vi "GFITS_ImlistMngr.vi"(6 "max bytes size":i32=200000, 8 "log":bool, 9 "arguments":string, 10 "command":string, 11 "images_witten_path":path=path "/home/ArcVIEW/Modules/Database/private/vis/imlist.log") -> (0 "log out":bool, 2 "answer":string)   [LabVIEW 2016]
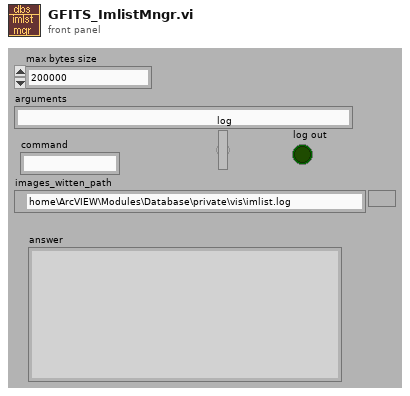
[diagram p1: front panel]
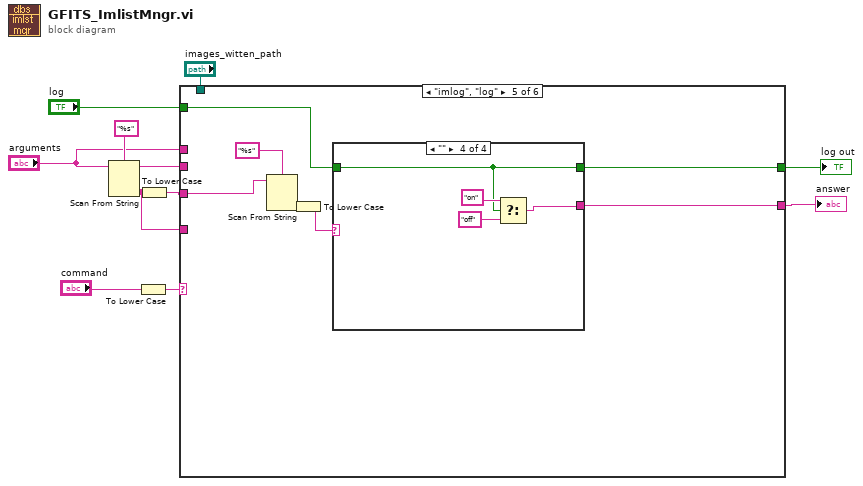
[diagram p0: block diagram]
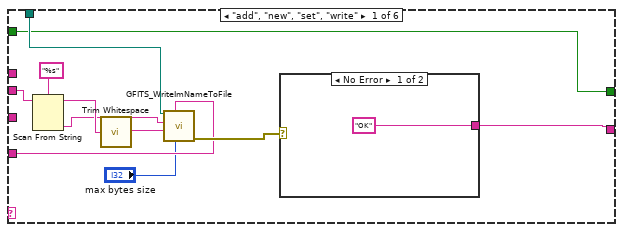
[diagram p2: hidden frame]
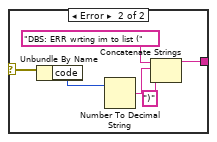
[diagram p3: hidden frame]
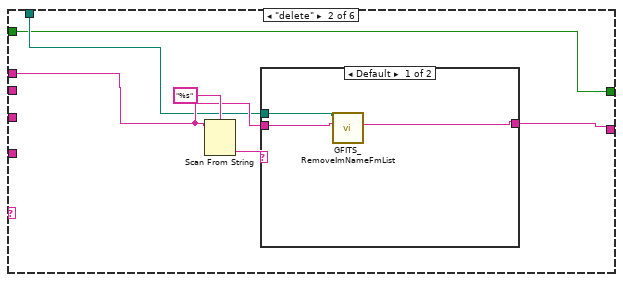
[diagram p4: hidden frame]
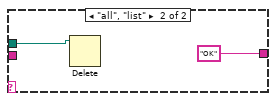
[diagram p5: hidden frame]
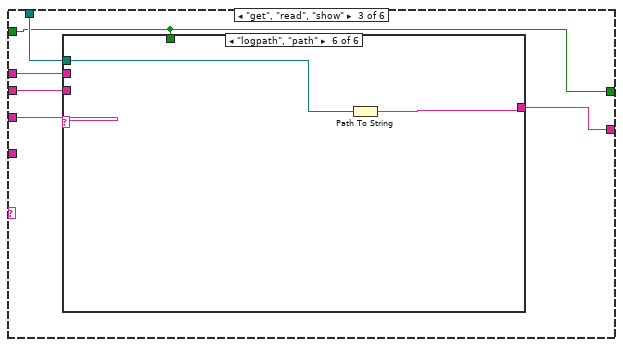
[diagram p6: hidden frame]
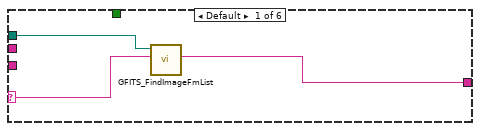
[diagram p7: hidden frame]
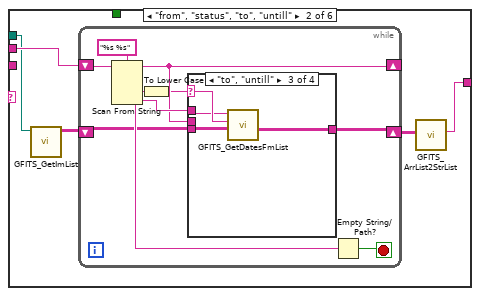
[diagram p8: hidden frame]
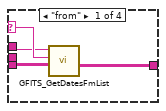
[diagram p9: hidden frame]
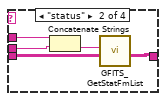
[diagram p10: hidden frame]
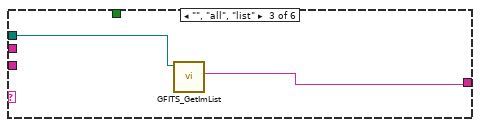
[diagram p12: hidden frame]
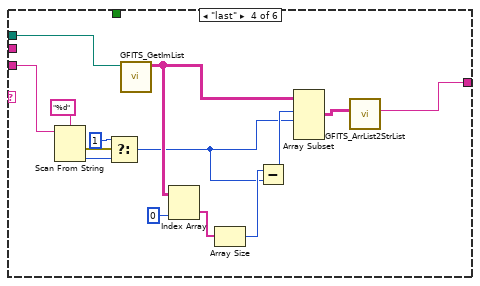
[diagram p13: hidden frame]
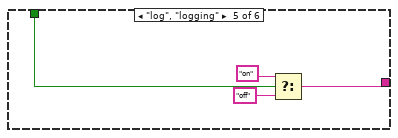
[diagram p14: hidden frame]
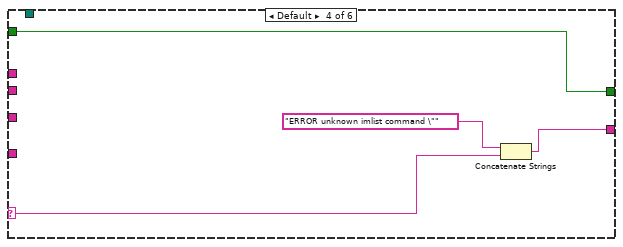
[diagram p15: hidden frame]
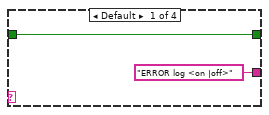
[diagram p16: hidden frame]
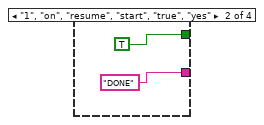
[diagram p17: hidden frame]
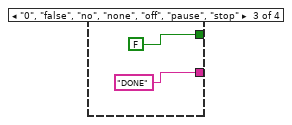
[diagram p18: hidden frame]
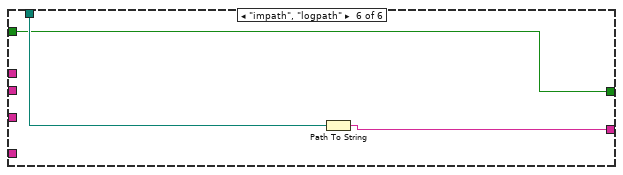
[diagram p19: hidden frame]
diagram:
  n1 = Scan From String(format string="%s", input string="arguments") -> (remaining string=w10:string, output 1=w3:string)  [unwired: 2 in, 3 out]
  n2 = To Lower Case(string="command") -> (all lower case string=w7:string)
  n3 = To Lower Case(string=w3) -> (all lower case string=w5:string)
  n4 = case shown="\"imlog\", \"log\"" w7 {
    selector: w7 -> [_ _ _ w102 _ _]
    tunnel: w5 -> [_ _ w46 _ w104 _]
    tunnel: w10 -> [w20 _ w45 _ _ _]
    tunnel: "images_witten_path" -> [w13 w31 w42 _ _ w123]
    tunnel: [w21 w35 w44 w101 w106 w122] -> w9
    tunnel: "arguments" -> [_ w32 w43 _ _ _]
    tunnel: w3 -> [w15 _ _ _ _ _]
    tunnel: "log" -> [w12 w30 w41 w100 w105 w121]
    tunnel: [w12 w30 w41 w100 w107 w121] -> w1
    frame "add", "new", "set", "write" {
      n5 = Scan From String(format string="%s", input string=w20) -> (remaining string=w18:string, output 1=w16:string)  [unwired: 2 in, 3 out]
      n6 = call <vilib>:"Trim Whitespace.vi"("string"=w18) -> ("trimmed string"=w17:string)  [unwired: 1 in]
      n7 = call "GFITS_WriteImNameToFile.vi"("max bytes size"="max bytes size", "id"=w15, "Status"=w17, "Image"=w16, "Path"=w13) -> ("error out"=w22:errorcluster)  [unwired: 1 in, 5 out]
      n8 = case shown="No Error" w22 {
        selector: w22 -> [_ w28]
        tunnel: ["OK" w24] -> w21
        frame No Error {
        }
        frame Error {
          n9 = Unbundle By Name(w28) -> ("code"=w27:i32)
          n10 = Number To Decimal String(number=w27) -> (decimal integer string=w26:string)  [unwired: 1 out]
          n11 = Concatenate Strings("DBS: ERR wrting im to list (", w26, ")" ("string")) -> (w24:string)
        }
      }
    }
    frame "delete" {
      n12 = Scan From String(format string="%s", input string=w32) -> (output 1=w33:string)  [unwired: 2 in, 4 out]
      n13 = case shown="Default" w33 {
        tunnel: [w36 "OK" ("answer")] -> w35
        tunnel: w31 -> [w38 w39]
        tunnel: w32 -> [w37 _]
        frame Default {
          n14 = call "GFITS_RemoveImNameFmList.vi"("Image"=w37, "Path"=w38) -> ("answer"=w36:string)  [unwired: 2 in, 7 out]
        }
        frame "all", "list" {
          n15 = Delete(path (use dialog)=w39) -> ()  [unwired: 1 in, 6 out]
        }
      }
    }
    frame "get", "read", "show" {
      n16 = case shown="\"logpath\", \"path\"" w46 {
        selector: w46 -> [w47 _ _ _ _ _]
        tunnel: w45 -> [_ _ _ w92 _ _]
        tunnel: [w48 w50 w78 w80 w95 w98] -> w44
        tunnel: w42 -> [w49 w53 w79 w93 _ w99]
        tunnel: w43 -> [_ w54 _ _ _ _]
        tunnel: w41 -> [_ _ _ _ w97 _]
        frame Default {
          n17 = call "GFITS_FindImageFmList.vi"("Image"=w47, "Path"=w49) -> ("status"=w48:string)  [unwired: 1 in, 8 out]
        }
        frame "from", "status", "to", "untill" {
          n18 = call "GFITS_GetImList.vi"("Path"=w53) -> ("list"=w52:string[][])  [unwired: 1 in, 9 out]
          n19 = while {
            shift-right: [w56] -> _
            shift-left: w54 -> [w63]
            shift-right: [w57] -> w51
            shift-left: w52 -> [w58]
            stop <- w59 stop-if-true
            n20 = Scan From String(format string="%s %s", input string=w63) -> (remaining string=w56:string, output 1=w61:string, output 2=w60:string)  [unwired: 2 in, 4 out]
            n21 = To Lower Case(string=w61) -> (all lower case string=w55:string)
            n22 = case shown="\"to\", \"untill\"" w55 {
              selector: w55 -> [w65 _ w74 _]
              tunnel: w60 -> [w64 w70 w73 _]
              tunnel: w58 -> [w67 w72 w76 w77]
              tunnel: [w66 w71 w75 w77] -> w57
              tunnel: w56 -> [_ w69 _ _]
              frame "from" {
                n23 = call "GFITS_GetDatesFmList.vi"("List In"=w67, "action"=w65, "timestamp"=w64) -> ("List Out"=w66:string[][])  [unwired: 8 out]
              }
              frame "status" {
                n24 = Concatenate Strings(w70, w69) -> (w68:string)
                n25 = call "GFITS_GetStatFmList.vi"("List In"=w72, "status"=w68) -> ("List Out"=w71:string[][])  [unwired: 9 out]
              }
              frame "to", "untill" {
                n26 = call "GFITS_GetDatesFmList.vi"("List In"=w76, "action"=w74, "timestamp"=w73) -> ("List Out"=w75:string[][])  [unwired: 8 out]
              }
              frame Default {
              }
            }
            n27 = Empty String/Path?(string/path=w60) -> (empty?=w59:bool)
          }
          n28 = call "GFITS_ArrList2StrList.vi"("List In"=w51) -> ("List Out"=w50:string)  [unwired: 9 out]
        }
        frame "", "all", "list" {
          n29 = call "GFITS_GetImList.vi"("Path"=w79) -> ("answer"=w78:string)  [unwired: 1 in, 9 out]
        }
        frame "last" {
          n30 = Scan From String(format string="%d", input string=w92) -> (error out=w90:errorcluster, output 1=w89:i32)  [unwired: 2 in, 3 out]
          n31 = Select(t=1, s=w90, f=w89) -> (s? t:f=w82:i32)
          n32 = call "GFITS_GetImList.vi"("Path"=w93) -> ("list"=w85:string[][])  [unwired: 1 in, 9 out]
          n33 = Index Array(array=w85, index (col)=0 ("disabled index (col)")) -> (element=w86:string[])  [unwired: 1 in]
          n34 = Array Size(array=w86) -> (size(s)=w84:i32)
          n35 = Subtract(x=w84, y=w82) -> (x-y=w83:i32)
          n36 = Array Subset(array=w85, index (row)=w83, length (row)=w82) -> (w81:string[][])  [unwired: 2 in]
          n37 = call "GFITS_ArrList2StrList.vi"("List In"=w81) -> ("List Out"=w80:string)  [unwired: 9 out]
        }
        frame "log", "logging" {
          n38 = Select(t="on", s=w97, f="off") -> (s? t:f=w95:string)
        }
        frame "logpath", "path" {
          n39 = Path To String(path=w99) -> (string=w98:string)
        }
      }
    }
    frame Default {
      n40 = Concatenate Strings("ERROR unknown imlist command \"" ("answer"), w102) -> (w101:string)
    }
    frame "imlog", "log" {
      n41 = Scan From String(format string="%s", input string=w104) -> (output 1=w109:string)  [unwired: 2 in, 4 out]
      n42 = To Lower Case(string=w109) -> (all lower case string=w108:string)
      n43 = case shown="\"\"" w108 {
        tunnel: [w111 TRUE ("log") FALSE ("log") w118] -> w107
        tunnel: ["ERROR log <on |off>" ("List Out") "DONE" ("List Out") "DONE" ("List Out") w117] -> w106
        tunnel: w105 -> [w111 _ _ w118]
        frame Default {
        }
        frame "1", "on", "resume", "start", "true", "yes" {
        }
        frame "0", "false", "no", "none", "off", "pause", "stop" {
        }
        frame "" {
          n44 = Select(t="on", s=w118, f="off") -> (s? t:f=w117:string)
        }
      }
    }
    frame "impath", "logpath" {
      n45 = Path To String(path=w123) -> (string=w122:string)
    }
  }
  "answer" <- w9
  "log out" <- w1
